vi "Wf binary to float.vi"(2 "Input string":string) -> (16 "Data out":dbl[](array[numeric]))   [LabVIEW 2010, in "RedPitaya.lvlib"]
uses:
  RedPitaya.lvlib
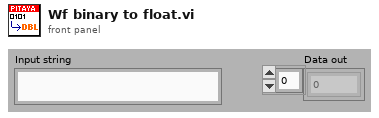
[diagram p1: front panel]
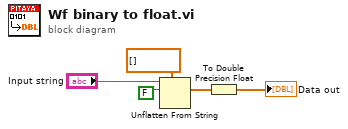
[diagram p0: block diagram]
diagram:
  n1 = Unflatten From String(type=sgl[] [] ("Si"), binary string="Input string", data includes array or string size? (T)=FALSE) -> (value=w2:sgl[])  [unwired: 2 in, 2 out]
  n2 = To Double Precision Float(number=w2) -> (double precision float=→"Data out":dbl[])
